vi "GEA2 Send Message.vi"(0 "GEA2 Reference In":refnum<k24>, 1 "Input Data":T1 {"Command" format="%02x"; "Destination" format="%02x"; "Source" format="%02x"}, 2 "Retry Count":u32=3, 11 "Error In":errorcluster) -> (4 "GEA2 Reference Out":refnum<k24>, 15 "Error Out":errorcluster)   [LabVIEW 2014, in "GEA2_Toolkit.lvlib"]
doc: "This VI sends a GEA2 message accross the GEA2 bus."
uses:
  library/GEA2_Toolkit.lvlib
  C:/Automation/DLLs/PC Tools .NET/GeaCommunication.dll
  Automation/DLLs/PC Tools .NET/GeaCommunication.dll
  type defs/Data In.ctl
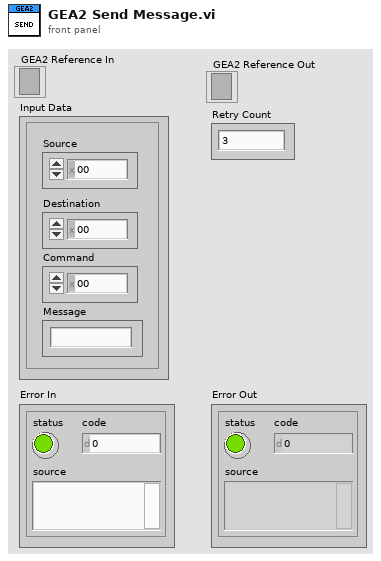
[diagram p1: front panel]
types:
  T1 = typedef "GEA2_Toolkit.lvlib/Data In.ctl" = cluster{"Source":u8, "Destination":u8, "Command":u8, "Message":string}
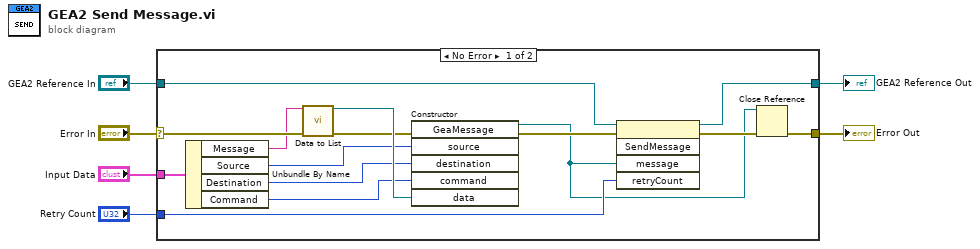
[diagram p0: block diagram]
diagram:
  n1 = case shown="No Error" "Error In" {
    selector: "Error In" -> [w18 w22]
    tunnel: "GEA2 Reference In" -> [w7 w23]
    tunnel: [w17 w23] -> w3
    tunnel: [w13 w22] -> w5
    tunnel: "Retry Count" -> [w16 _]
    tunnel: "Input Data" -> [w12 _]
    frame No Error {
      n2 = Unbundle By Name(w12) -> ("Message"=w10:string, "Source"=w11:u8, "Destination"=w9:u8, "Command"=w8:u8)
      n3 = call "Data to List.vi"("Data String In"=w10, "error in"=w18) -> ("Data List Out"=w20:refnum<k24>, "error out"=w19:errorcluster)  [unwired: 12 in]
      n4 = constructor class="GeaMessage"(error in=w19, "source"=w11, "destination"=w9, "command"=w8, "data"=w20) -> (reference out=w14:refnum<k24>, error out=w21:errorcluster)  [unwired: 2 in, 5 out]
      n5 = invoke method="SendMessage"(reference=w7, error in=w21, "message"=w14, "retryCount"=w16) -> (reference out=w17:refnum<k24>, error out=w15:errorcluster)  [unwired: 1 in, 3 out]
      n6 = Close Reference(reference=w14, error in (no error)=w15) -> (error out=w13:errorcluster)
    }
    frame Error {
    }
  }
  "Error Out" <- w5
  "GEA2 Reference Out" <- w3
